vi "Configure System.vi"(0 "VISA resource name":refnum<visa-resource-name>, 1 "Unit Address (1)":i16=1, 2 "Power-Out Time (10.0)":dbl=10.0 format="%.2f", 3 "Power-Out Action (0: Continue)":u16(ring) items=["Continue", "Hold", "Terminate", "Reset", "Idle Set Point 1", "Idle Set Point 2"], 5 "PID Units (0: US)":u16(ring) items=["US", "SI"], 7 "Temperature Scale (0: °F)":u16(ring) items=["°F", "°C"], 9 "Show °C or °F (T: Yes)":bool=TRUE, 11 "error in (no error)":errorcluster {"code" format="%.0x"}) -> (4 "VISA resource name out":refnum<visa-resource-name>, 15 "error out":errorcluster {"code" format="%.0x"})   [LabVIEW 2010]
doc: "This VI defines the global operating characteristics of the controller."
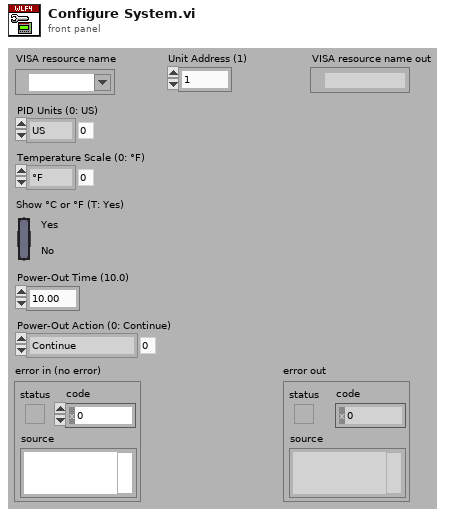
[diagram p1: front panel]
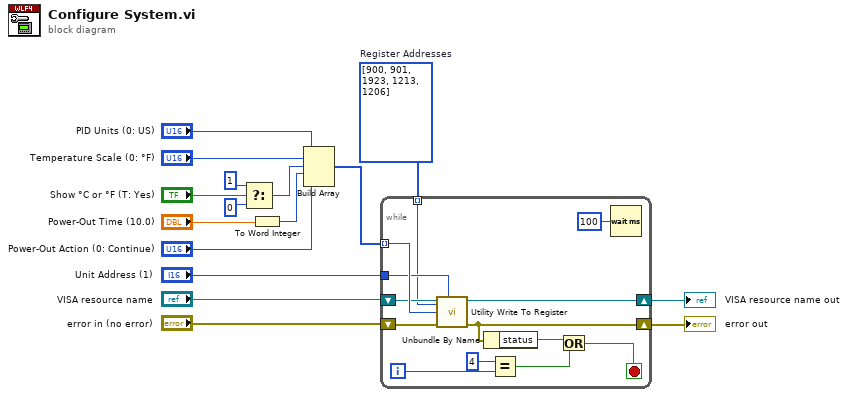
[diagram p0: block diagram]
diagram:
  w8 = i32[] [900, 901, 1923, 1213, 1206]  # Register Addresses
  n1 = Select(t=i16 1, s="Show °C or °F (T: Yes)", f=i16 0) -> (s? t:f=w4:i16)
  n2 = To Word Integer(number="Power-Out Time (10.0)") -> (16bit integer=w1:i16)
  n3 = Build Array("PID Units (0: US)", "Temperature Scale (0: °F)", w4, w1, "Power-Out Action (0: Continue)") -> (w9:u16[])
  n4 = while {
    tunnel: w9 -> [w29] mode=indexing
    tunnel: "Unit Address (1)" -> [w28]
    shift-right: [w25] -> w14
    shift-left: "VISA resource name" -> [w27]
    shift-right: [w22] -> w13
    shift-left: "error in (no error)" -> [w26]
    tunnel: w8 -> [w23] mode=indexing
    i -> [w19]
    stop <- w20 stop-if-true
    n5 = call "Utility Write To Register.vi"("Unit Address (1)"=w28, "error in (no error)"=w26, "Data (0)"=w29, "Register Address (0)"=w23, "VISA resource name"=w27) -> ("error out"=w22:errorcluster, "VISA resource name out"=w25:refnum<visa-resource-name>)  [unwired: 5 in]
    n6 = Unbundle By Name(w22) -> ("status"=w21:bool)
    n7 = Equal?(x=4, y=w19) -> (x = y?=w17:bool)
    n8 = Or(x=w21, y=w17) -> (x .or. y?=w20:bool)
    n9 = Wait (ms)(milliseconds to wait=u32 100) -> ()  [unwired: 1 out]
  }
  "error out" <- w13
  "VISA resource name out" <- w14
